vi "Close Path Associated Instruments.vi"(0 "Path Groups in":refnum<class "Path Group.lvclass">[](array[class]), 11 "error in":errorcluster) -> (4 "Path Groups out":refnum<class "Path Group.lvclass">[](array[class]), 15 "error out":errorcluster)   [LabVIEW 2023, in "RFFixtureCharact.Public.lvlib"]
uses:
  RFFixtureCharact.Public.lvlib
  Common/Base Classes/Path Group/Path Group.lvclass
  Common/RFCalAndFixtureCharact.Common.lvlib
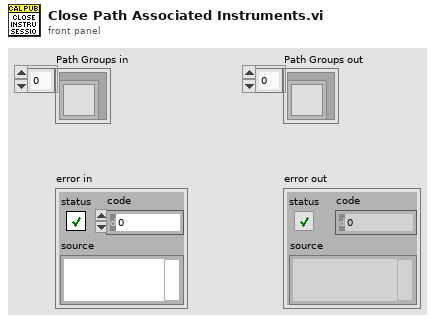
[diagram p1: front panel]
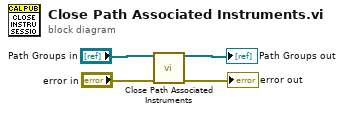
[diagram p0: block diagram]
diagram:
  n1 = call "Close Path Associated Instruments.vi"("Path Groups in"="Path Groups in", "error in (no error)"="error in") -> ("Path Groups out"=→"Path Groups out":refnum<class "Path Group.lvclass">[], "error out"=→"error out":errorcluster)  [unwired: 12 in]
